vi "Collect.vi"(6 "error in":errorcluster, 9 "FlatSequenceFrame in":refnum<class "FlatSequenceFrame.lvclass">) -> (0 "error out":errorcluster, 3 "FlatSequenceFrame out":refnum<class "FlatSequenceFrame.lvclass">, 4 "collect":string)   [LabVIEW 2014, in "FlatSequenceFrame.lvclass"]
uses:
  FlatSequenceFrame.lvclass
  Python/Parsing/ListTypesTD.ctl
  FlatSequenceFrame.lvclass/FlatSequenceFrame.ctl
  FlatSequenceOuterTunnel/FlatSequenceOuterTunnel.lvclass/FlatSequenceOuterTunnel.ctl
  FlatSequenceInnerTunnel/FlatSequenceInnerTunnel.lvclass/FlatSequenceInnerTunnel.ctl
  Terminal/Terminal.lvclass
  Python/Parsing/Python Functions.lvlib
  FlatSequenceInnerTunnel/FlatSequenceInnerTunnel.lvclass
  FlatSequenceOuterTunnel/FlatSequenceOuterTunnel.lvclass
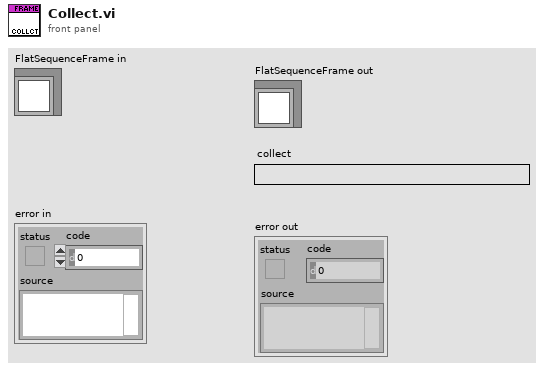
[diagram p1: front panel]
types:
  T1 = typedef "Python Functions.lvlib/ListTypesTD.ctl" = enum16{"list", "tuple", "parameter list", "output list"}
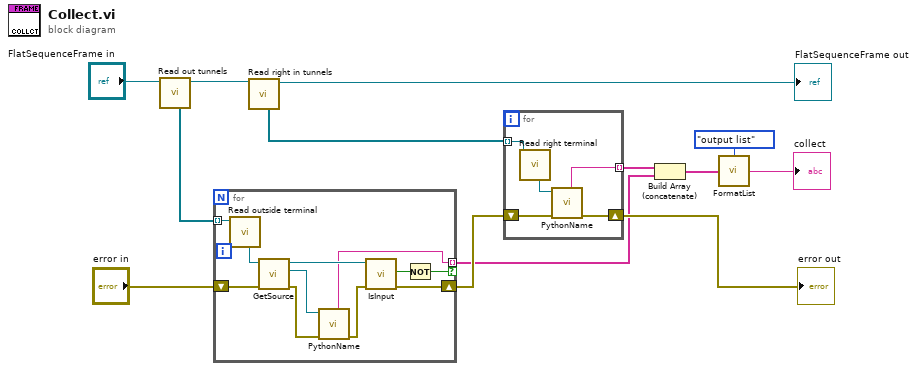
[diagram p0: block diagram]
diagram:
  n1 = call "Read out tunnels.vi"("FlatSequenceFrame in"="FlatSequenceFrame in") -> ("FlatSequenceFrame out"=w8:refnum<class "FlatSequenceFrame.lvclass">, "out tunnels"=w12:refnum<class "FlatSequenceOuterTunnel.lvclass">[])  [unwired: 7 in]
  n2 = for {
    tunnel: w12 -> [w24] mode=indexing
    tunnel: [w14] -> w1 mode=indexing if=w21
    shift-right: [w23] -> w3
    shift-left: "error in" -> [w18]
    n3 = call "Read outside terminal.vi"("FlatSequenceInnerTunnel in"=w24) -> ("outside terminal"=w20:refnum<class "Terminal.lvclass">)  [unwired: 7 in, 1 out]
    n4 = call "GetSource.vi"("error in"=w18, "Terminal in"=w20) -> ("error out"=w17:errorcluster, "source"=w16:refnum<class "Terminal.lvclass">, "Terminal out"=w19:refnum<class "Terminal.lvclass">)  [unwired: 5 in]
    n5 = call-dynamic "PythonName.vi"("error in"=w17, "Terminal in"=w16) -> ("error out"=w15:errorcluster, "name"=w14:string)  [unwired: 6 in, 2 out]
    n6 = call-dynamic "IsInput.vi"("error in"=w15, "Terminal in"=w19) -> ("error out"=w23:errorcluster, "input"=w22:bool)  [unwired: 5 in, 1 out]
    n7 = Not(x=w22) -> (.not. x?=w21:bool)
  }
  n8 = call "Read right in tunnels.vi"("FlatSequenceFrame in"=w8) -> ("FlatSequenceFrame out"=→"FlatSequenceFrame out":refnum<class "FlatSequenceFrame.lvclass">, "right in tunnels"=w9:refnum<class "FlatSequenceInnerTunnel.lvclass">[])  [unwired: 7 in]
  n9 = for {
    tunnel: [w27] -> w11 mode=indexing
    tunnel: w9 -> [w29] mode=indexing
    shift-right: [w25] -> w2
    shift-left: w3 -> [w26]
    n10 = call "Read right terminal.vi"("FlatSequenceInnerTunnel in"=w29) -> ("right terminal"=w28:refnum<class "Terminal.lvclass">)  [unwired: 7 in, 1 out]
    n11 = call-dynamic "PythonName.vi"("error in"=w26, "Terminal in"=w28) -> ("error out"=w25:errorcluster, "name"=w27:string)  [unwired: 6 in, 2 out]
  }
  "error out" <- w2
  n12 = Build Array (concatenate)(w11, w1) -> (w10:string[])
  n13 = call "FormatList.vi"("values"=w10, "type"=ListTypesTD."output list") -> ("python object"=→"collect":string)
